vi "ql2_response_to_id.vi"(11 "response_type":T1) -> (2 "query_type_ids":u32[](array[numeric]), 3 "id":u32)   [LabVIEW 2017, in "rethinkdb.lvlib"]
uses:
  rethinkdb.lvlib
  ql2_response.ctl
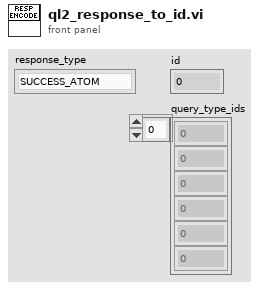
[diagram p1: front panel]
types:
  T1 = typedef "rethinkdb.lvlib/ql2_response.ctl" = enum8{"SUCCESS_ATOM", "SUCCESS_SEQUENCE", "SUCCESS_PARTIAL", "WAIT_COMPLETE", "SERVER_INFO", "CLIENT_ERROR", "COMPILE_ERROR", "RUNTIME_ERROR", "invalid"}
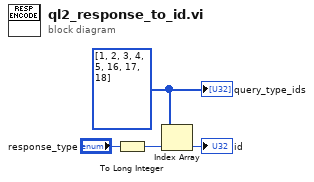
[diagram p0: block diagram]
diagram:
  w1 = u32[] [1, 2, 3, 4, 5, 16, 17, 18] ("ids")
  n1 = To Long Integer(number="response_type") -> (32bit integer=w3:i32)
  n2 = Index Array(array=w1, index=w3) -> (element=→"id":u32)
  "query_type_ids" <- w1
